vi "dfd_Dummy_FIRMultiplyUnit.vi"(0 "opState":T1, 2 "x(n)":fxp<+/-,64,32>, 3 "coef":fxp<+/-,16,1>) -> (4 "x(n-1)":fxp<+/-,64,32>, 7 "y(n)":fxp<+/-,64,32>)   [LabVIEW 2017]
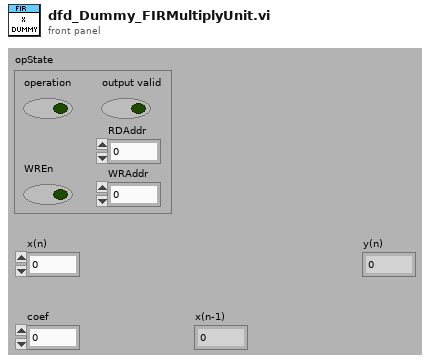
[diagram p1: front panel]
types:
  T1 = cluster{"operation":bool, "RDAddr":u16, "WREn":bool, "WRAddr":u16, "output valid":bool}
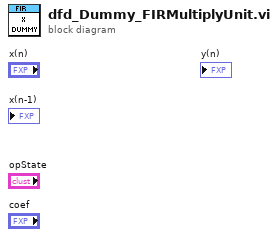
[diagram p0: block diagram]
diagram:
